vi "MED_AMPL_EX.vi"(11 "path":path) -> ()   [LabVIEW 2009]
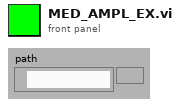
[diagram p1: front panel]
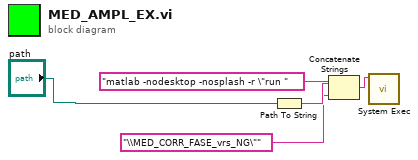
[diagram p0: block diagram]
diagram:
  n1 = Path To String(path="path") -> (string=w4:string)
  n2 = Concatenate Strings("matlab -nodesktop -nosplash -r \"run " ("command line"), w4, "\\MED_CORR_FASE_vrs_NG\"" ("command line")) -> (w3:string)
  n3 = call <vilib>:"System Exec.vi"("command line"=w3) -> ()  [unwired: 7 in, 4 out]
